vi "GoogleMapsAPI_V2009.vi"() -> ()   [LabVIEW 2011]
panel:
  in  "stop":bool
  in  "Google Maps API Key":string
  in  "Show Path?":bool=TRUE
  in  "Weight":i32=5
  in  "Path Collor":u32(colorbox)=16715776
  in  "character":string="a"
  in  "color":string(combo)="purple"
  in  "size":string(combo)="mid"
  in  "Longitude":dbl=-1.307 format="%#.6g"
  in  "Latitude":dbl=51.4062 format="%#.6g"
  in  "Map Format":string(combo)="hybrid"
  in  "X":dbl=350.0
  in  "Y":dbl=570.0
  in  "Zoom":sgl=18.0 format="%#.1g"
  in  "Lon":dbl=-1.3070000000000026 format="%#.6g"
  in  "Lat":dbl=51.4062 format="%#.6g"
  out "URL":string="http://maps.google.com/staticmap?center=51.406200,-1.307000&zoom=18&size=570x350&maptype=hybrid&markers=51.406200,-1.307000,midpurplea&key=&path=rgb:0xFF1000,weight:5|51.406200,-1.307000|51.406200,-1.307000"
  in  "?":refnum<k7>(container)
  # "Start Position"
  # "Balloon Position"
  # "This is an 86 character alphanumeric key supplied by Google"
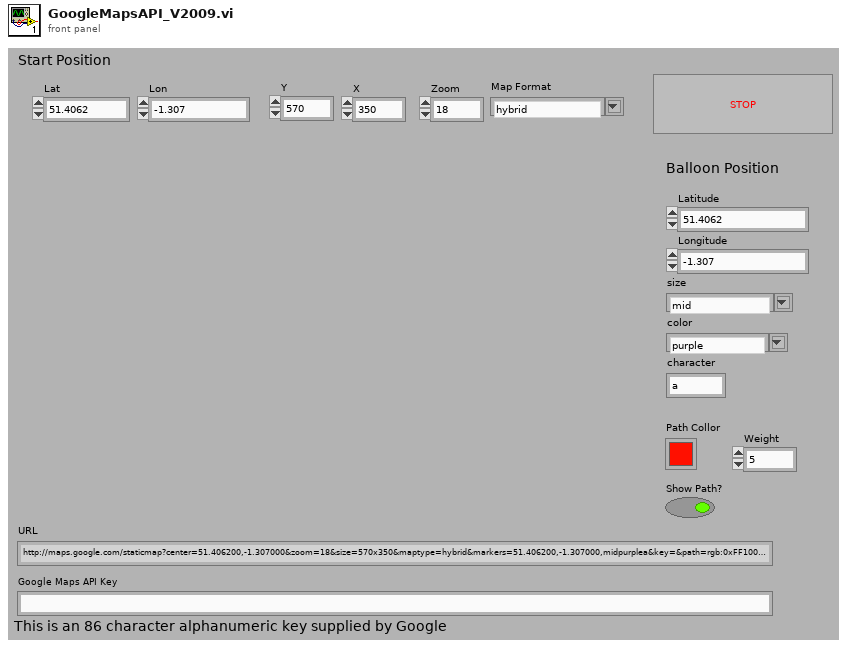
[diagram p1: front panel]
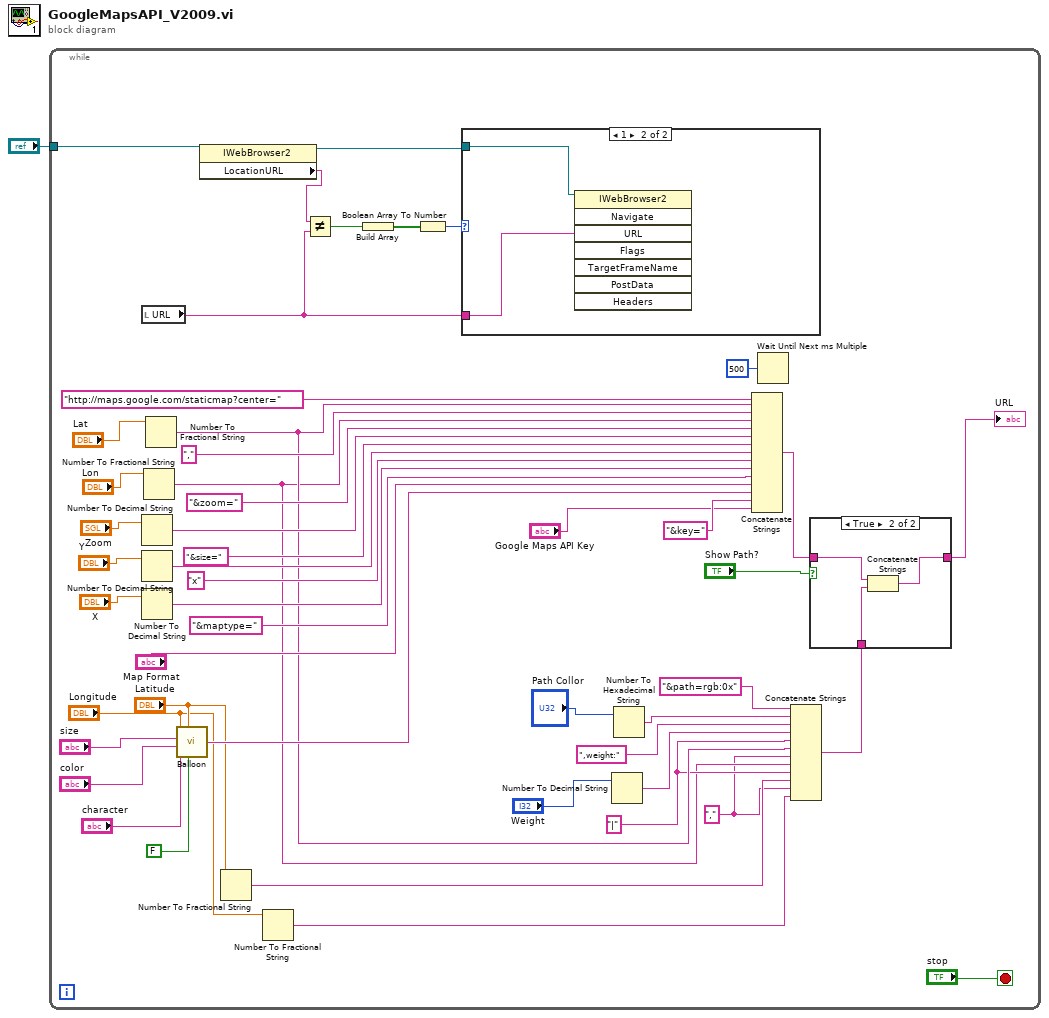
[diagram p0: block diagram]
diagram:
  n1 = while {
    tunnel: "?" -> [w49]
    stop <- "stop" stop-if-true
    w7 = "," ("string")
    w9 = "|"
    n2 = local read "URL"() -> (w43:string)
    n3 = Number To Decimal String(number="Zoom") -> (decimal integer string=w36:string)  [unwired: 1 in]
    n4 = Number To Decimal String(number="Y") -> (decimal integer string=w32:string)  [unwired: 1 in]
    n5 = Number To Decimal String(number="X") -> (decimal integer string=w30:string)  [unwired: 1 in]
    n6 = Number To Fractional String(number="Lon") -> (F-format string=w8:string)  [unwired: 3 in]
    n7 = Number To Fractional String(number="Lat") -> (F-format string=w16:string)  [unwired: 3 in]
    n8 = call "Balloon.vi"("One more?"=FALSE, "Latitude"="Latitude", "character"="character", "color"="color", "size"="size", "Longitude"="Longitude") -> ("Balloon"=w27:string)
    n9 = property class="IWebBrowser2"(reference=w49) -> (reference out=w48:refnum<k7>, "LocationURL"=w46:string)  [unwired: 1 in, 1 out]
    n10 = Number To Fractional String(number="Latitude") -> (F-format string=w10:string)  [unwired: 3 in]
    n11 = Number To Fractional String(number="Longitude") -> (F-format string=w11:string)  [unwired: 3 in]
    n12 = Not Equal?(x=w46, y=w43) -> (x != y?=w47:bool)
    n13 = Build Array(w47) -> (w45:bool[])
    n14 = Boolean Array To Number(Boolean array=w45) -> (number=w44:u32)
    n15 = case shown="1" w44 {
      tunnel: w43 -> [_ w56]
      tunnel: w48 -> [_ w55]
      frame 0, Default {
      }
      frame 1 {
        n16 = invoke class="IWebBrowser2" method="Navigate"(reference=w55, "URL"=w56) -> ()  [unwired: 6 in, 8 out]
      }
    }
    n17 = Number To Decimal String(number="Weight") -> (decimal integer string=w17:string)  [unwired: 1 in]
    n18 = Number To Hexadecimal String(2:"Path Collor") -> (0:w20:string)  [unwired: 1 in]
    n19 = Concatenate Strings("http://maps.google.com/staticmap?center=" ("URL"), w16, "," ("string"), w8, "&zoom=", w36, "&size=", w32, "x", w30, "&maptype=", "Map Format", w27, "&key=" ("string"), "Google Maps API Key") -> (w12:string)
    n20 = Wait Until Next ms Multiple(millisecond multiple=u32 500) -> ()  [unwired: 1 out]
    n21 = Concatenate Strings("&path=rgb:0x" ("string"), w20, ",weight:", w17, w9, w16, w7, w8, w9, w10, w7, w11) -> (w14:string)
    n22 = case shown="True" "Show Path?" {
      tunnel: w14 -> [_ w54]
      tunnel: [w51 w53] -> w13
      tunnel: w12 -> [w51 w52]
      frame False {
      }
      frame True {
        n23 = Concatenate Strings(w52, w54) -> (w53:string)
      }
    }
    "URL" <- w13
  }
